vi "Initialize Transfer Group.vi"(5 "FIFO Options":T1, 7 "id":i32, 8 "error in (no error)":errorcluster, 9 "force inline? (F)":bool, 10 "Transfer Group Buffers":refnum<class "Buffers.lvclass">, 11 "Transfer Group Configuration":T2={"name"="", "direction"=enum."Tx", "cycle timing"={"priority"=0, "decimation"=1, "offset"=0}, "thread"=-1, "settings"=[], "Transfers"=[]} {"Transfers"."channels"."string descriptor"."buffer offset" format="%d bytes"; "Transfers"."channels"."engine descriptor"."buffer offset" format="%d bytes"}) -> (0 "error out":errorcluster, 3 "Transfer Group out":refnum<class "Transfer Group.lvclass">)   [LabVIEW 2017, in "DSF Core.lvlib" / "Transfer Group.lvclass"]
uses:
  Transfer Group.lvclass
  DSF Configuration API/Public/Controls/DSF Engine Transfer Group Configuration.ctl
  DSF Configuration API/Public/Controls/DSF Direction.ctl
  DSF Configuration API/Public/Controls/DSF Timing Info.ctl
  DSF Configuration API/Public/Controls/DSF Settings Info.ctl
  DSF Configuration API/Public/Controls/DSF Engine Transfer Configuration.ctl
  DSF Configuration API/Public/Controls/DSF Byte Order.ctl
  DSF Configuration API/Public/Controls/DSF Engine Channel Configuration.ctl
  DSF Configuration API/Public/Controls/DSF Channel Buffer Descriptor.ctl
  DSF Configuration API/Public/Controls/DSF Data Type.ctl
  Buffer/Buffers.lvclass
  Typedefs/FIFO Flags.ctl
  Shared/VIs/Sizeof.vi
  DSF Configuration API/Public/Required String Buffer Size (Transfer).vi
  DSF Configuration API/Public/Channel Count (Transfer).vi
  Transfer/Transfer.lvclass
  DSF Core.lvlib
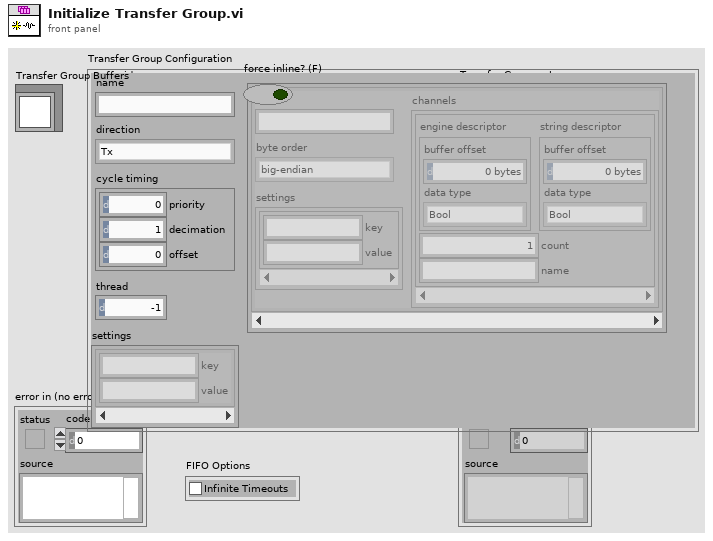
[diagram p1: front panel]
types:
  T1 = typedef "DSF Core.lvlib/FIFO Flags.ctl" = cluster{"Infinite Timeouts":bool}
  T2 = typedef "DSF Core.lvlib/DSF Engine Transfer Group Configuration.ctl" = cluster{"name":string, "direction":T3, "cycle timing":T4, "thread":i32, "settings":T5, "Transfers":T6[]}
  T3 = typedef "DSF Core.lvlib/DSF Direction.ctl" = enum8{"Tx", "Rx"}
  T4 = typedef "DSF Core.lvlib/DSF Timing Info.ctl" = cluster{"priority":u64, "decimation":u64, "offset":u64}
  T5 = typedef "DSF Core.lvlib/DSF Settings Info.ctl" = cluster{"key":string, "value":string}[]
  T6 = typedef "DSF Core.lvlib/DSF Engine Transfer Configuration.ctl" = cluster{"name":string, "byte order":T7, "channels":T8[], "settings":T5}
  T7 = typedef "DSF Core.lvlib/DSF Byte Order.ctl" = enum8{"big-endian", "little-endian"}
  T8 = typedef "DSF Core.lvlib/DSF Engine Channel Configuration.ctl" = cluster{"engine descriptor":T9, "string descriptor":T9, "count":u64, "name":string}
  T9 = typedef "DSF Core.lvlib/DSF Channel Buffer Descriptor.ctl" = cluster{"buffer offset":u64, "data type":T10}
  T10 = typedef "DSF Core.lvlib/DSF Data Type.ctl" = enum8{"Bool", "SGL", "DBL", "I8", "I16", "I32", "I64", "U8", "U16", "U32", "U64"}
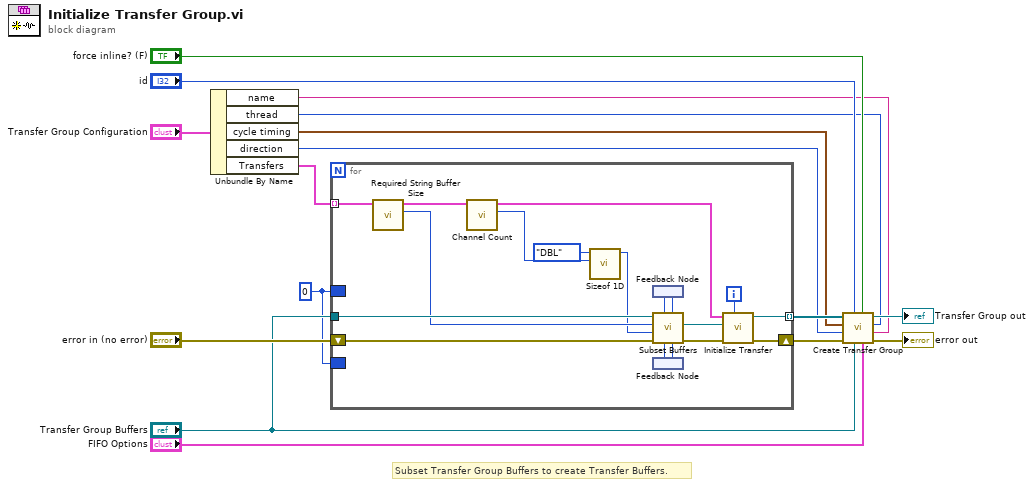
[diagram p0: block diagram]
diagram:
  w6 = u64 0 ("inline buffer size")
  # "Subset Transfer Group Buffers to create Transfer Buffers."
  n1 = Unbundle By Name("Transfer Group Configuration") -> ("name"=w1:string, "thread"=w2:i32, "cycle timing"=w10:T4, "direction"=w9:T3, "Transfers"=w13:T6[])
  n2 = for {
    tunnel: w13 -> [w31] mode=indexing
    tunnel: [w34] -> w11 mode=indexing
    shift-right: [w33] -> w12
    shift-left: "error in (no error)" -> [w26]
    border: w6 -> [_]
    border: w6 -> [_]
    tunnel: "Transfer Group Buffers" -> [w25]
    i -> [w32]
    n3 = call-poly "Required String Buffer Size.vi"("Transfer Configuration in"=w31) -> ("required string buffer size"=w18:u64, "Transfer Configuration out"=w30:T6)  [unwired: 8 in, 1 out]
    n4 = call-poly "Channel Count.vi"("Transfer Configuration in"=w30) -> ("total channel count"=w28:u64, "Transfer Configuration out"=w29:T6)  [unwired: 8 in, 1 out]
    n5 = call "Sizeof 1D.vi"("count"=w28, "data type"=DSF_Data_Type."DBL") -> ("size in bytes"=w17:u64)  [unwired: 9 in]
    n6 = feedback #1() -> (w22:u64)
    n7 = feedback #2() -> (w24:u64)
    n8 = call "Subset Buffers.vi"("inline buffer offset"=w24, "string buffer offset"=w22, "error in (no error)"=w26, "inline buffer size"=w17, "string buffer size"=w18, "Buffers in"=w25) -> ("error out"=w20:errorcluster, "subset Buffers"=w19:refnum<class "Buffers.lvclass">, "inline buffer offset +size"=w23:u64, "string buffer offset + size"=w21:u64)  [unwired: 1 in, 1 out]
    n9 = feedback-in #1(w21) -> ()
    n10 = feedback-in #2(w23) -> ()
    n11 = call "Initialize Transfer.vi"("id"=w32, "error in (no error)"=w20, "Buffers"=w19, "Transfer Configuration"=w29) -> ("error out"=w33:errorcluster, "Transfer out"=w34:refnum<class "Transfer.lvclass">)  [unwired: 6 in]
  }
  n12 = call "Create Transfer Group.vi"("name"=w1, "thread"=w2, "FIFO Options"="FIFO Options", "force inline? (F)"="force inline? (F)", "Buffers"="Transfer Group Buffers", "id"="id", "error in (no error)"=w12, "direction"=w9, "cycle timing"=w10, "Transfers"=w11) -> ("error out"=→"error out":errorcluster, "Transfer Group out"=→"Transfer Group out":refnum<class "Transfer Group.lvclass">)
